vi "Get max counts all cameras.vi"() -> ()   [LabVIEW 2020]
panel:
  out "HighCountsCams":string[](array[string])
  out "Array":dbl[](array[numeric])
  out "variable value":string
  out "timed out":bool
  out "error out":errorcluster
  out "Device name":string
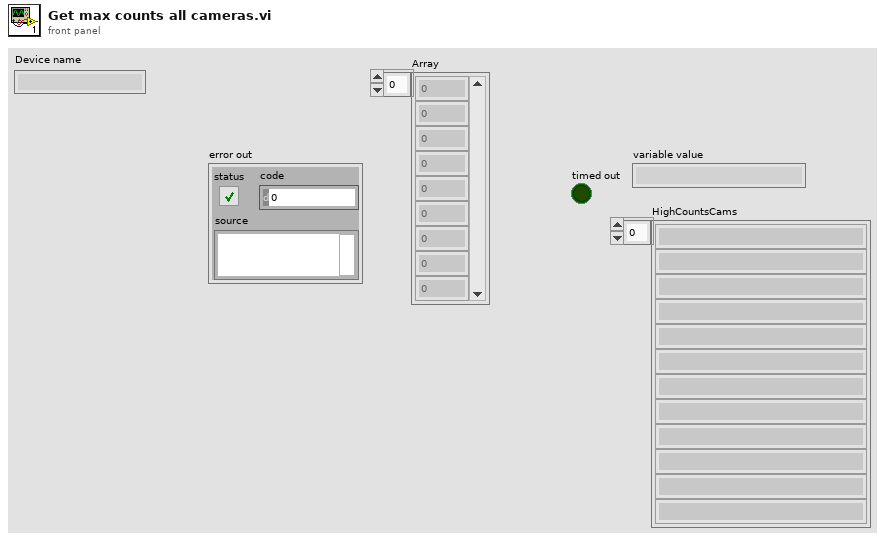
[diagram p1: front panel]
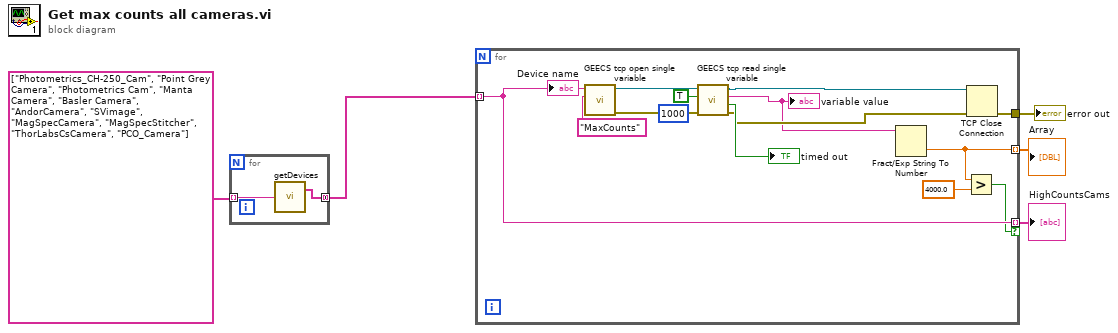
[diagram p0: block diagram]
diagram:
  n1 = for {
    tunnel: [w7] -> w3 mode=concatenating
    tunnel: string[] ["Photometrics_CH-250_Cam", "Point Grey Camera", "Photometrics Cam", "Manta Camera", "Basler Camera", "AndorCamera", "SVimage", "MagSpecCamera", "MagSpecStitcher", "ThorLabsCsCamera", "PCO_Camera"] -> [w6] mode=indexing
    n2 = call "getDevices.vi"("Device Class"=w6) -> ("All Devices"=w7:string[])  [unwired: 1 out]
  }
  n3 = for {
    tunnel: [w20] -> w4
    tunnel: w3 -> [w11] mode=indexing
    tunnel: [w10] -> w2 mode=indexing
    tunnel: [w11] -> w1 mode=indexing if=w8
    n4 = call "GEECS tcp open single variable.vi"("Variable name"="MaxCounts", "Device name"=w11) -> ("error out"=w16:errorcluster, "TCP Network Connection out"=w17:refnum<k5>)  [unwired: 7 in, 1 out]
    n5 = call "GEECS tcp read single variable.vi"("error in (no error)"=w16, "timeout ms (2000)"=1000, "clear buffer after read"=TRUE, "TCP Network Connection in"=w17) -> ("error out"=w14:errorcluster, "timed out"=→"timed out":bool, "variable value"=w13:string, "TCP Network Connection out"=w15:refnum<k5>)  [unwired: 4 in]
    "variable value" <- w13
    n6 = Fract/Exp String To Number(string=w13) -> (number=w10:dbl)  [unwired: 3 in, 1 out]
    n7 = Greater?(x=w10, y=4000.0) -> (0:w8:bool)
    n8 = TCP Close Connection(connection ID=w15, error in (no error)=w14) -> (error out=w20:errorcluster)  [unwired: 1 in, 1 out]
    "Device name" <- w11
  }
  "error out" <- w4
  "Array" <- w2
  "HighCountsCams" <- w1
